vi "saverunnumber.vi"(9 "RunNumber":u16=4, 11 "VI path":path) -> ()   [LabVIEW 2020]
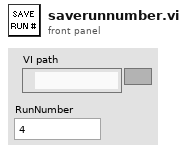
[diagram p1: front panel]
types:
  T1 = enum16{"open", "replace", "create", "open or create", "replace or create", "replace or create with confirmation"}
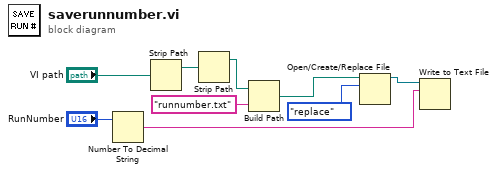
[diagram p0: block diagram]
diagram:
  n1 = Number To Decimal String(number="RunNumber") -> (decimal integer string=w3:string)  [unwired: 1 in]
  n2 = Strip Path(path="VI path") -> (stripped path=w9:path)  [unwired: 1 out]
  n3 = Strip Path(path=w9) -> (stripped path=w8:path)  [unwired: 1 out]
  n4 = Build Path(base path=w8, name or relative path="runnumber.txt") -> (appended path=w6:path)
  n5 = Open/Create/Replace File(file path (use dialog)=w6, operation (0:open)=T1."replace") -> (refnum out=w4:refnum<file>)  [unwired: 4 in, 2 out]
  n6 = Write to Text File(file (use dialog)=w4, text=w3) -> ()  [unwired: 2 in, 3 out]
